vi "Big Endian to Little Endian string.vi"(11 "Input (Big Endian)":string) -> (3 "Output (Little Endian)":string)   [LabVIEW 2020, in "Library Commun.lvlib"]
uses:
  Library Commun.lvlib
panel:
  # "This VI invert the input in Big Endian plain string to Little Endian plain string"
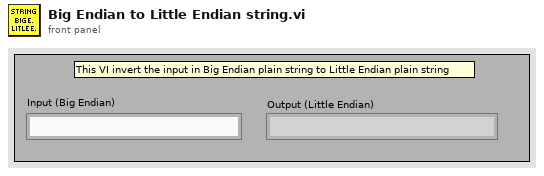
[diagram p1: front panel]
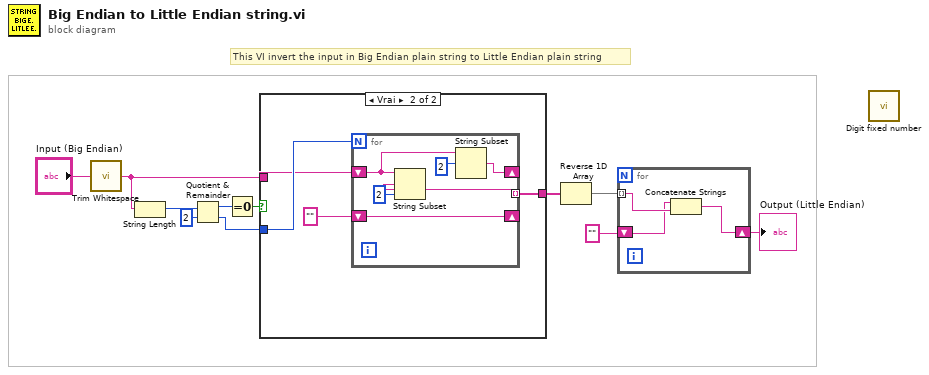
[diagram p0: block diagram]
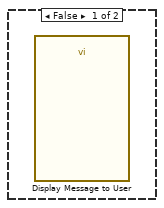
[diagram p2: hidden frame]
diagram:
  # "This VI invert the input in Big Endian plain string to Little Endian plain string"
  n1 = call <vilib>:"Trim Whitespace.vi"("string"="Input (Big Endian)") -> ("trimmed string"=w8:string)  [unwired: 1 in]
  n2 = String Length(string=w8) -> (length=w6:i32)
  n3 = Quotient & Remainder(x=w6, y=2) -> (x-y*floor(x/y)=w9:i32, floor(x/y)=w5:i32)
  n4 = Equal To 0?(x=w9) -> (x = 0?=w7:bool)
  n5 = case shown="Vrai" w7 {
    tunnel: w8 -> [_ w13]
    tunnel: w5 -> [_ w15]
    tunnel: [_ w12] -> w4
    frame False {
      n6 = call "Display Message to User"() -> ()  [unwired: 10 in, 2 out]
    }
    frame True {
      n7 = for {
        N: w15 -> [_]
        shift-right: [w21] -> _
        shift-left: "" -> [w21]
        shift-right: [w16] -> _
        shift-left: w13 -> [w18]
        tunnel: [w19] -> w12 mode=indexing
        n8 = String Subset(string=w18, length (rest)=2 ("length (rest)")) -> (substring=w19:string)  [unwired: 1 in]
        n9 = String Subset(string=w18, offset (0)=2 ("length (rest)")) -> (substring=w16:string)  [unwired: 1 in]
      }
    }
  }
  n10 = Reverse 1D Array(array=w4) -> (reversed array=w3:string[])
  n11 = for {
    tunnel: w3 -> [w23] mode=indexing
    shift-right: [w24] -> w1
    shift-left: "" -> [w22]
    n12 = Concatenate Strings(w22, w23) -> (w24:string)
  }
  "Output (Little Endian)" <- w1
  n13 = call "Digit fixed number.vi"() -> ()  [unwired: 11 in, 1 out]
